vi "Cross_spectra_and_phase.vi"(0 "U1":dbl[](array[numeric]) format="%.2f", 2 "U2":dbl[](array[numeric]) format="%.2f") -> (5 "U1 spectra":cluster{dbl, dbl, dbl[]}(graph), 6 "U2 spectra":cluster{dbl, dbl, dbl[]}(graph), 7 "U1 U2 coherence":cluster{dbl, dbl, "Coherence array":dbl[]}(graph), 8 "U1 U2 phase":cluster{dbl, dbl, "Phase array":dbl[]}(graph))   [LabVIEW 2020]
doc: "This VI produces ensemble-averaged spectra, coherence and phase outputs for a pair of similarly sampled signals.\nThe outputs are single-sided, and commence at 1.dF, the 0Hz term having been removed."
uses:
  Globals/Meas_global.vi
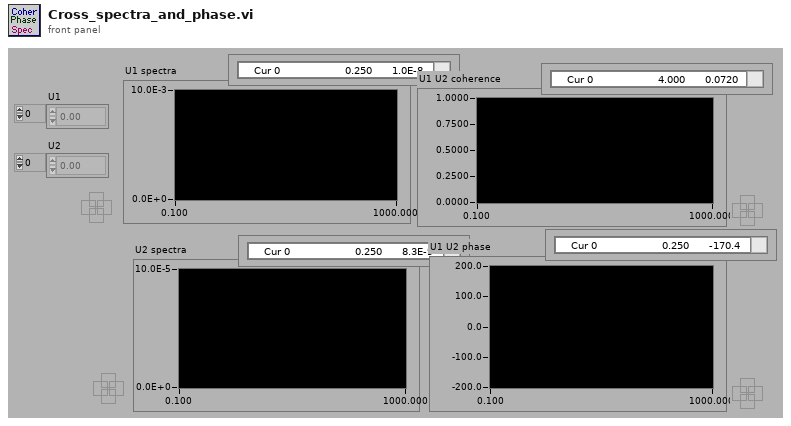
[diagram p1: front panel]
types:
  T1 = typedef "Analysis_info_cluster.ctl" = cluster{"Colour":u32, "Inst type":T2, "Inst name":string, "Symbol":string, "Code name":string, "Extra Info":string, "Inst Array":T3, "Extra Titles":string[], "Extra Values":string[], "U":dbl, "u^2":dbl, "u^3":dbl, "u^4":dbl, "Skew_u":dbl, "Kurt_u":dbl, "Sd Error in Mean":dbl, "% u'/U":dbl, "X":dbl, "Y":dbl, "Z":dbl, "Timescale integral Estimate":dbl, "Sd Error in Variance":dbl, "Calib File":path, "Calib Constants":dbl[], "Output Position":bool, "Stats":enum16{"None", "Basic", "Full"}, "Av Sampling Rate":dbl, "Av No of Samples":dbl, "Total Meas Time (s)":dbl, "ADAM Ch Name":string, "Max value":dbl, "Min value":dbl, "Req Sample Rate Hz":dbl, "Sync Delay Time (s)":dbl, "Ch No":i16, "Device":string, "Use Latest Calib":bool, "Port":string, "Metadata Ch Names":string[], "Metadata Ch Values":string[], "Label":string}
  T2 = typedef "Inst_type.ctl" = enum16{"Raw voltage", "Raw with zero offsetting", "Propeller anemometer", "Pressure Transducer", "Pitot-static tube", "Hot wire", "Cross wire 1", "Cross wire 2", "Generic Linear", "Generic Polynomial", "Generic BackPoly", "Fast FID", "Thermocouple", "Cold wire", "Pulsed Wire", "LDA Vel", "LDA Tran time", "LDA Arr time", "Microphone"}
  T3 = typedef "Instrument_Array.ctl" = enum16{"PWA", "LDA", "Analogue"}
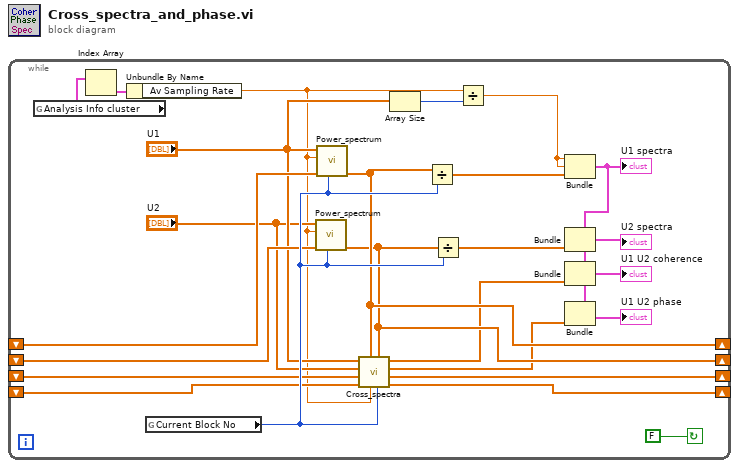
[diagram p0: block diagram]
diagram:
  n1 = while {
    shift-left: _ -> [w21]
    shift-right: [w19] -> _
    shift-left: _ -> [w22]
    shift-right: [w20] -> _
    shift-left: _ -> [w23]
    shift-right: [w17] -> _
    shift-left: _ -> [w24]
    shift-right: [w18] -> _
    stop <- FALSE continue-if-true
    n2 = global read "Meas_global.vi" "Analysis Info cluster"() -> (w3:T1[])
    n3 = Index Array(array=w3) -> (element=w2:T1)  [unwired: 1 in]
    n4 = Unbundle By Name(w2) -> ("Av Sampling Rate"=w1:dbl)
    n5 = global read "Meas_global.vi" "Current Block No"() -> (w25:i32)
    n6 = call "Power_spectrum.vi"("Block No"=w25, "Spectrum input array"=w23, "Sampling frequency"=w1, "U"="U2") -> ("Spectrum Accumulator array"=w17:dbl[])  [unwired: 1 in, 3 out]
    n7 = call "Power_spectrum.vi"("Block No"=w25, "Spectrum input array"=w24, "Sampling frequency"=w1, "U"="U1") -> ("Spectrum Accumulator array"=w18:dbl[])  [unwired: 1 in, 3 out]
    n8 = call "Cross_spectra.vi"("block number"=w25, "S11 input array"=w17, "sampling frequency"=w1, "S22 input array"=w18, "Im(S12) input array"=w21, "Re(S12) input array"=w22, "U2"="U2", "U1"="U1") -> ("Im(S12) output array"=w19:dbl[], "Re(S12) output array"=w20:dbl[], "Phase array"=w12:dbl[], "Coherence array"=w13:dbl[])
    n9 = Array Size(array="U1") -> (size(s)=w11:i32)
    n10 = Divide(x=w18, y=w25) -> (x/y=w15:dbl[])
    n11 = Divide(x=w17, y=w25) -> (x/y=w14:dbl[])
    n12 = Divide(x=w1, y=w11) -> (x/y=w6:dbl)
    n13 = Bundle(w6, w6, w15) -> (w7:cluster{dbl, dbl, dbl[]})  [unwired: 1 out]
    "U1 spectra" <- w7
    n14 = Bundle(cluster=w7, w14) -> (→"U2 spectra":cluster{dbl, dbl, dbl[]})  [unwired: 2 out]
    n15 = Bundle(cluster=w7, w13) -> (→"U1 U2 coherence":cluster{dbl, dbl, dbl[]})  [unwired: 2 out]
    n16 = Bundle(cluster=w7, w12) -> (→"U1 U2 phase":cluster{dbl, dbl, dbl[]})  [unwired: 2 out]
  }
